vi "Agilent SNA Format Model String.vi"(1 "Model String":string) -> (0 "Model":T1)   [LabVIEW 2011]
uses:
  TypeDefs/Agilent SNA Model.ctl
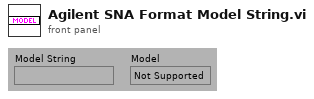
[diagram p1: front panel]
types:
  T1 = typedef "Agilent SNA Model.ctl" = enum16{"Not Supported", "8757X"}
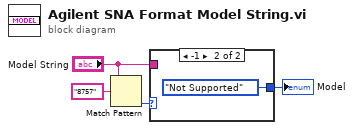
[diagram p0: block diagram]
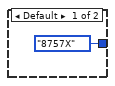
[diagram p2: hidden frame]
diagram:
  n1 = Match Pattern(string="Model String", regular expression="8757") -> (offset past match=w2:i32)  [unwired: 4 out]
  n2 = case shown="-1" w2 {
    tunnel: "Model String" -> [_ _]
    tunnel: [Agilent_SNA_Model."8757X" ("Model") Agilent_SNA_Model."Not Supported" ("Model")] -> w4
    frame Default {
    }
    frame -1 {
    }
  }
  "Model" <- w4
